vi "Average Waveforms By RMS.vi"(8 "error in":errorcluster, 9 "Result Live Graph Plotter in":refnum<class "Live Graph Plotter.lvclass">, 10 "Waveforms Selection":T1={"Record Start Index (0)"=0, "Record Length (-1)"=-1, "Channel List (All)"=""}, 11 "Original Live Graph Plotter in":refnum<class "Live Graph Plotter.lvclass">) -> (0 "error out":errorcluster, 1 "Result Live Graph Plotter out":refnum<class "Live Graph Plotter.lvclass">)   [LabVIEW 2025]
doc: "Average waveforms by RMS"
uses:
  Live Graph Plotter/Live Graph Plotter.lvclass
  <vilib>/Analysis/NI_AALPro.lvlib
  <vilib>/Analysis/5stat.llb/RMS (DBL).vi
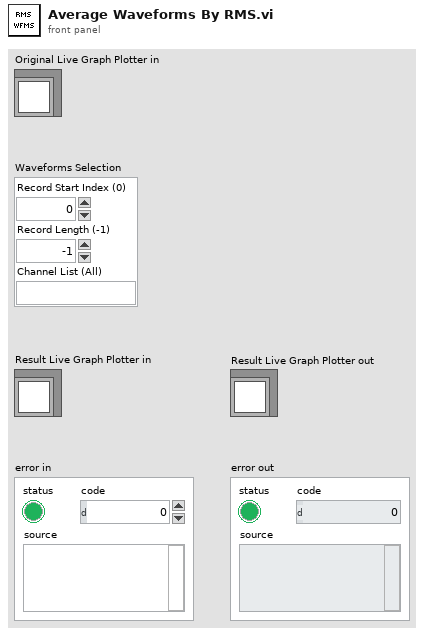
[diagram p1: front panel]
types:
  T1 = cluster{"Record Start Index (0)":i32, "Record Length (-1)":i32, "Channel List (All)":string}
  T2 = cluster{"Channel Name":string, "relativeInitialX":dbl, "xIncrement":dbl, "Waveforms":cluster{"wfm":dbl[]}[]}[]
  T3 = cluster{"relativeInitialX":dbl, "xIncrement":dbl, dbl[]}
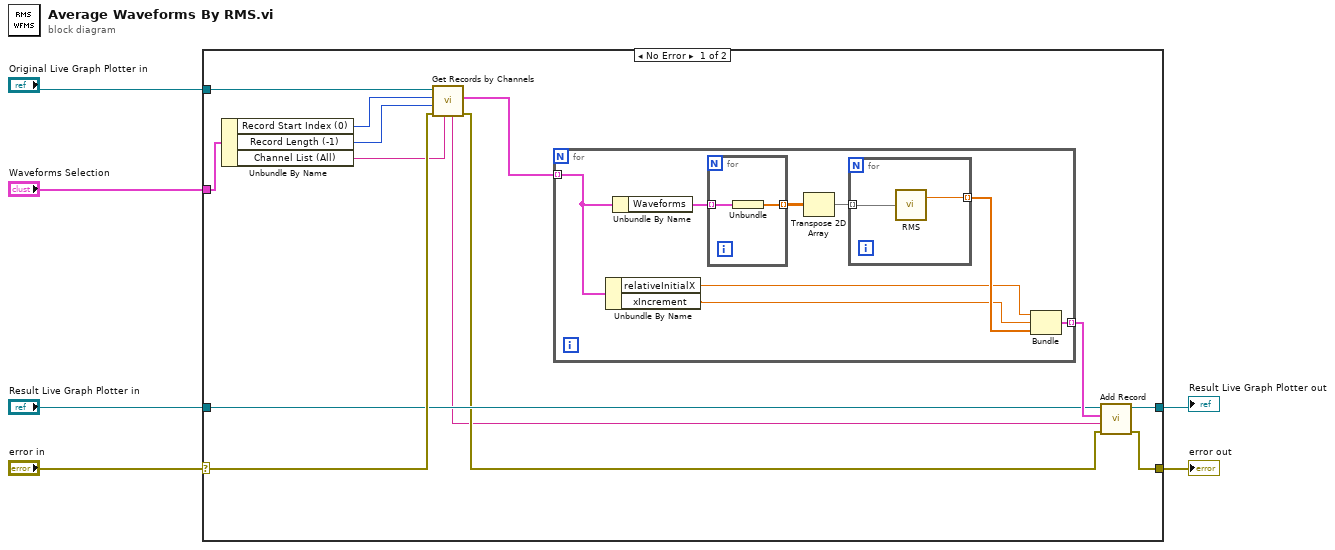
[diagram p0: block diagram]
diagram:
  n1 = case shown="No Error" "error in" {
    selector: "error in" -> [w18 w32]
    tunnel: "Original Live Graph Plotter in" -> [w19 _]
    tunnel: [w8 w32] -> w4
    tunnel: "Waveforms Selection" -> [w17 _]
    tunnel: "Result Live Graph Plotter in" -> [w11 w33]
    tunnel: [w10 w33] -> w1
    frame No Error {
      n2 = Unbundle By Name(w17) -> ("Record Start Index (0)"=w16:i32, "Record Length (-1)"=w13:i32, "Channel List (All)"=w12:string)
      n3 = call "Get Records by Channels.vi"("Channel List (All)"=w12, "error in (no error)"=w18, "Record Length (-1)"=w13, "Record Start Index (0)"=w16, "Live Graph Plotter in"=w19) -> ("error out"=w9:errorcluster, "Records By Channels"=w15:T2, "Channel List"=w7:string)  [unwired: 3 in, 1 out]
      n4 = for {
        tunnel: w15 -> [w23] mode=indexing
        tunnel: [w20] -> w14 mode=indexing
        n5 = Unbundle By Name(w23) -> ("relativeInitialX"=w22:dbl, "xIncrement"=w21:dbl)
        n6 = Unbundle By Name(w23) -> ("Waveforms"=w27:cluster{"wfm":dbl[]}[])
        n7 = for {
          tunnel: w27 -> [w31] mode=indexing
          tunnel: [w30] -> w26 mode=indexing
          n8 = Unbundle(w31) -> ("wfm"=w30:dbl[])
        }
        n9 = Transpose 2D Array(2D array=w26) -> (transposed array=w25:dbl[][])
        n10 = for {
          tunnel: w25 -> [w29] mode=indexing
          tunnel: [w28] -> w24 mode=indexing
          n11 = call-poly <vilib>:"RMS.vi"("X"=w29) -> ("rms value"=w28:dbl)  [unwired: 1 out]
        }
        n12 = Bundle("relativeInitialX"=w22, "xIncrement"=w21, w24) -> (w20:T3)  [unwired: 1 in]
      }
      n13 = call "Add Record.vi"("error in (no error)"=w9, "Channel List"=w7, "Waveforms"=w14, "Live Graph Plotter in"=w11) -> ("error out"=w8:errorcluster, "Live Graph Plotter out"=w10:refnum<class "Live Graph Plotter.lvclass">)  [unwired: 6 in]
    }
    frame Error {
    }
  }
  "error out" <- w4
  "Result Live Graph Plotter out" <- w1
